vi "p07.vi"() -> ()   [LabVIEW 2015]
panel:
  out "number 6":u32
  out "number 5":u32
  out "number 4":u32
  out "number 3":u32
  out "number 2":u32
  out "number":u32
  out "U8":enum16{"s", "h", "r"}(ring)
  out "U32":enum16{"s", "h", "r"}(ring)
  out "U16":enum16{"s", "h", "r"}(ring)
  out "appended array":u32[](array[numeric])
  out "x .xor. y?":bool
  out "x .implies. y? 2":i32
  out "x .implies. y?":bool
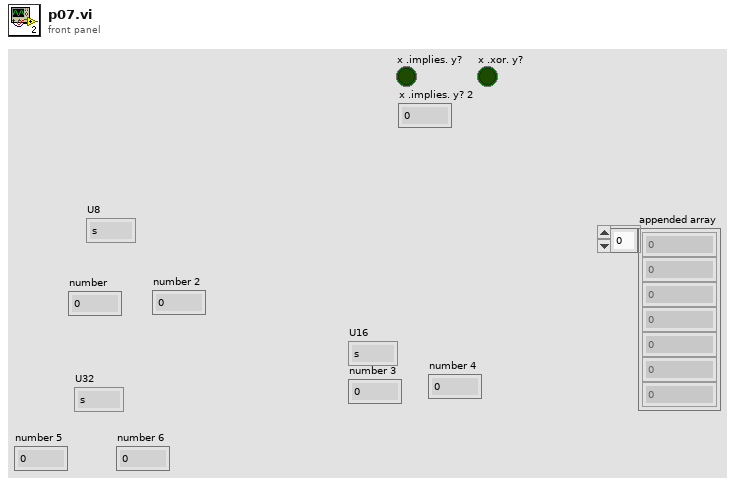
[diagram p1: front panel]
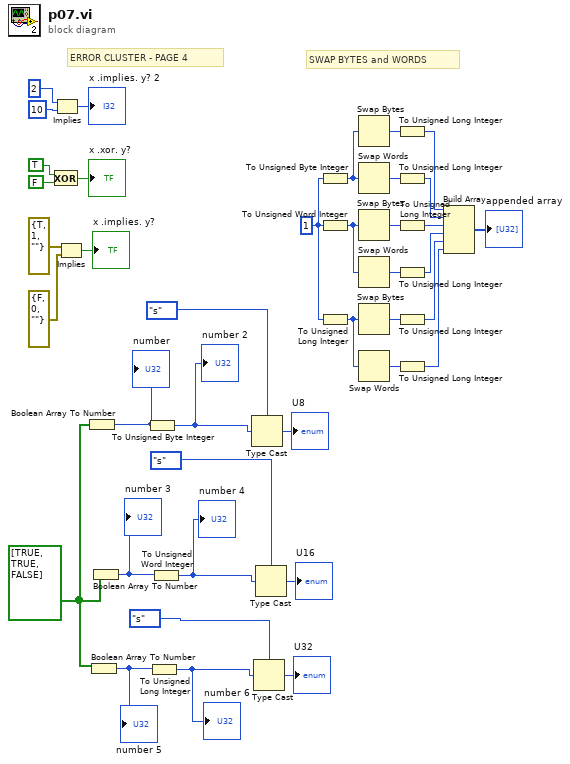
[diagram p0: block diagram]
diagram:
  w7 = bool[] [TRUE, TRUE, FALSE]
  w24 = 1 ("code")
  # "SWAP BYTES and WORDS"
  # "ERROR CLUSTER - PAGE 4"
  n1 = Exclusive Or(1:FALSE, 2:TRUE) -> (0:→"x .xor. y?":bool)
  n2 = Implies(1:10 ("code"), 2:2 ("code")) -> (0:→"x .implies. y? 2":i32)
  n3 = Implies(1:errorcluster {"status"=FALSE, "code"=0, "source"=""} ("y"), 2:errorcluster {"status"=TRUE, "code"=1, "source"=""} ("error constant")) -> (0:→"x .implies. y?":bool)
  n4 = Boolean Array To Number(Boolean array=w7) -> (number=w8:u32)
  "number" <- w8
  n5 = Boolean Array To Number(Boolean array=w7) -> (number=w1:u32)
  "number 5" <- w1
  n6 = Boolean Array To Number(Boolean array=w7) -> (number=w4:u32)
  "number 3" <- w4
  n7 = To Unsigned Byte Integer(number=w8) -> (unsigned 8bit integer=w5:u8)
  "number 2" <- w5
  n8 = To Unsigned Long Integer(number=w1) -> (unsigned 32bit integer=w2:u32)
  "number 6" <- w2
  n9 = To Unsigned Word Integer(number=w4) -> (unsigned 16bit integer=w3:u16)
  "number 4" <- w3
  n10 = Type Cast(type=enum16{"s", "h", "r", "e", "n", "i"}."s", x=w5) -> (*(type *) &x=→"U8":enum16{"s", "h", "r", "e", "n", "i"})
  n11 = Type Cast(type=enum16{"s", "h", "r", "e", "n", "i"}."s", x=w2) -> (*(type *) &x=→"U32":enum16{"s", "h", "r", "e", "n", "i"})
  n12 = Type Cast(type=enum16{"s", "h", "r", "e", "n", "i"}."s", x=w3) -> (*(type *) &x=→"U16":enum16{"s", "h", "r", "e", "n", "i"})
  n13 = To Unsigned Byte Integer(number=w24) -> (unsigned 8bit integer=w29:u8)
  n14 = To Unsigned Word Integer(number=w24) -> (unsigned 16bit integer=w25:u16)
  n15 = To Unsigned Long Integer(number=w24) -> (unsigned 32bit integer=w22:u32)
  n16 = Swap Bytes(anything=w29) -> (byte swapped=w30:u8)
  n17 = Swap Words(1:w29) -> (0:w28:u8)
  n18 = Swap Bytes(anything=w25) -> (byte swapped=w26:u16)
  n19 = Swap Words(1:w25) -> (0:w27:u16)
  n20 = Swap Bytes(anything=w22) -> (byte swapped=w23:u32)
  n21 = Swap Words(1:w22) -> (0:w21:u32)
  n22 = To Unsigned Long Integer(number=w30) -> (unsigned 32bit integer=w20:u32)
  n23 = To Unsigned Long Integer(number=w28) -> (unsigned 32bit integer=w19:u32)
  n24 = To Unsigned Long Integer(number=w26) -> (unsigned 32bit integer=w18:u32)
  n25 = To Unsigned Long Integer(number=w27) -> (unsigned 32bit integer=w17:u32)
  n26 = To Unsigned Long Integer(number=w23) -> (unsigned 32bit integer=w16:u32)
  n27 = To Unsigned Long Integer(number=w21) -> (unsigned 32bit integer=w15:u32)
  n28 = Build Array(w20, w19, w18, w17, w16, w15) -> (→"appended array":u32[])
